vi "Perform Action.vi"(8 "error in (no error)":errorcluster, 10 "Input":variant, 11 "Sample PID Watervalve in":refnum<class "Sample PID Watervalve.lvclass">) -> (0 "error out":errorcluster, 2 "Output":variant, 3 "Sample PID Watervalve out":refnum<class "Sample PID Watervalve.lvclass">)   [LabVIEW 2023, in "Sample PID Watervalve.lvclass"]
uses:
  Sample PID Watervalve.lvclass
  D:/git/HAL/HAL GOOP4/Task Base/Task Base.lvclass
  Task/Task Base/Task Base.lvclass/Task Base.ctl
  <vilib>/addons/control/pid/pid.llb/PID (DBL).vi
  Task/Task Base/Task Base.lvclass
  Measure and Stimulus Subsystems/Measure and Stimulus Subsystems.lvclass
  <vilib>/addons/control/pid/NI_PID_pid.lvlib
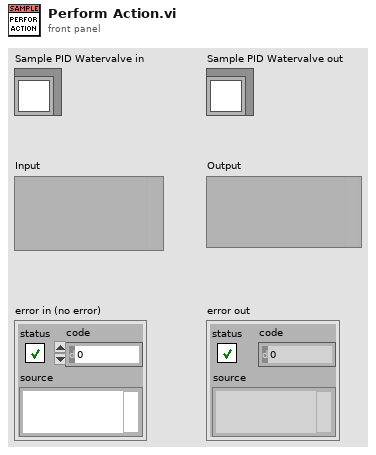
[diagram p1: front panel]
types:
  T1 = cluster{"Stop Notifier":refnum<notifier>, "Data Notifier":refnum<notifier>}
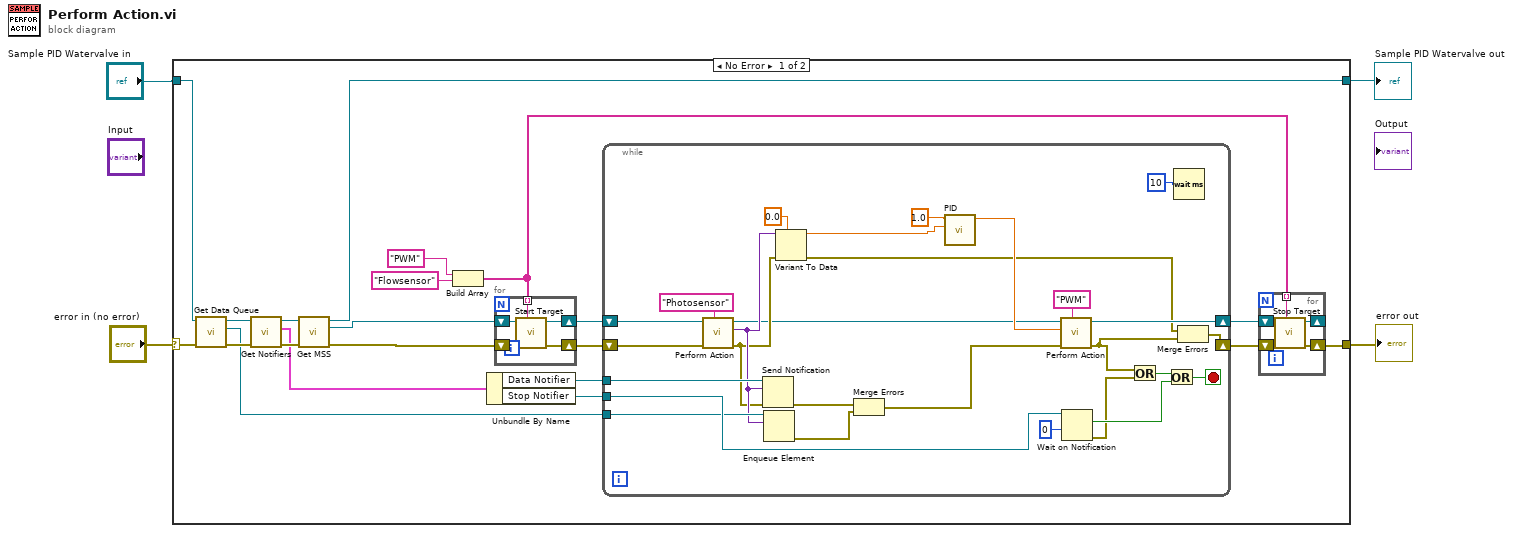
[diagram p0: block diagram]
diagram:
  n1 = case shown="No Error" "error in (no error)" {
    selector: "error in (no error)" -> [w22 w64]
    tunnel: [w18 w64] -> w1
    tunnel: [w5 w63] -> w2
    tunnel: "Sample PID Watervalve in" -> [w8 w63]
    frame No Error {
      n2 = call "Get Data Queue.vi"("error in (no error)"=w22, "Task Base in"=w8) -> ("error out"=w9:errorcluster, "Data Queue"=w6:refnum<queue>, "Task Base out"=w7:refnum<class "Sample PID Watervalve.lvclass">)  [unwired: 7 in]
      n3 = call "Get Notifiers.vi"("error in (no error)"=w9, "Task Base in"=w7) -> ("error out"=w17:errorcluster, "Notifier"=w13:T1, "Task Base out"=w16:refnum<class "Sample PID Watervalve.lvclass">)  [unwired: 7 in]
      n4 = call "Get MSS.vi"("error in (no error)"=w17, "Task Base in"=w16) -> ("error out"=w21:errorcluster, "MSS"=w20:refnum<class "Measure and Stimulus Subsystems.lvclass">, "Task Base out"=w5:refnum<class "Sample PID Watervalve.lvclass">)  [unwired: 7 in]
      n5 = Build Array("PWM" ("Target Ident"), "Flowsensor" ("Target Identifier")) -> (w10:string[])
      n6 = Unbundle By Name(w13) -> ("Data Notifier"=w11:refnum<notifier>, "Stop Notifier"=w12:refnum<notifier>)
      n7 = for {
        shift-right: [w30] -> w25
        shift-left: w21 -> [w28]
        shift-right: [w29] -> w24
        shift-left: w20 -> [w27]
        tunnel: w10 -> [w26] mode=indexing
        n8 = call "Start Target.vi"("Target Ident"=w26, "Error In"=w28, "reference in"=w27) -> ("Error Out"=w30:errorcluster, "reference out"=w29:refnum<class "Measure and Stimulus Subsystems.lvclass">)  [unwired: 7 in]
      }
      n9 = while {
        shift-right: [w48] -> w23
        shift-left: w25 -> [w53]
        shift-right: [w55] -> w19
        shift-left: w24 -> [w52]
        tunnel: w12 -> [w42]
        tunnel: w11 -> [w43]
        tunnel: w6 -> [w38]
        stop <- w46 stop-if-true
        n10 = call "Perform Action.vi"("Target Ident"="Photosensor" ("Target Identifier"), "Error In"=w53, "reference in"=w52) -> ("Error Out"=w32:errorcluster, "Output"=w33:variant, "reference out"=w31:refnum<class "Measure and Stimulus Subsystems.lvclass">)  [unwired: 6 in]
        n11 = Send Notification(notification=w33, notifier=w43, error in (no error)=w32) -> (error out=w35:errorcluster)  [unwired: 1 out]
        n12 = Enqueue Element(queue=w38, element=w33) -> (error out=w37:errorcluster)  [unwired: 2 in, 2 out]
        n13 = Variant To Data(error in=w32, type=0.0, Variant=w33) -> (data=w50:dbl, error out=w47:errorcluster)
        n14 = Merge Errors(w35, w37) -> (w36:errorcluster)
        n15 = call-poly <vilib>:"PID.vi"("process variable"=w50, "setpoint"=1.0) -> ("output"=w49:dbl)  [unwired: 8 in, 1 out]
        n16 = call "Perform Action.vi"("Target Ident"="PWM", "Error In"=w36, "Input"=w49, "reference in"=w31) -> ("Error Out"=w39:errorcluster, "reference out"=w55:refnum<class "Measure and Stimulus Subsystems.lvclass">)  [unwired: 5 in, 1 out]
        n17 = Wait on Notification(notifier=w42, timeout in ms (-1)=0) -> (notification=w44:bool, error out=w41:errorcluster)  [unwired: 2 in, 2 out]
        n18 = Or(x=w39, y=w41) -> (x .or. y?=w40:bool)
        n19 = Or(x=w40, y=w44) -> (x .or. y?=w46:bool)
        n20 = Wait (ms)(milliseconds to wait=u32 10) -> ()  [unwired: 1 out]
        n21 = Merge Errors(w47, w39) -> (w48:errorcluster)
      }
      n22 = for {
        shift-right: [w60] -> w18
        shift-left: w23 -> [w62]
        tunnel: w10 -> [w59] mode=indexing
        shift-right: [w58] -> _
        shift-left: w19 -> [w61]
        n23 = call "Stop Target.vi"("Target Ident"=w59, "Error In"=w62, "reference in"=w61) -> ("Error Out"=w60:errorcluster, "reference out"=w58:refnum<class "Measure and Stimulus Subsystems.lvclass">)  [unwired: 7 in]
      }
    }
    frame Error {
    }
  }
  "error out" <- w1
  "Sample PID Watervalve out" <- w2
